vi "test Import Same Module Different Configuration.vi"(8 "error in (no error)":errorcluster, 11 "TestCase in":refnum<class "SLSC Switch Import Unit Tests.lvclass">) -> (0 "error out":errorcluster, 3 "TestCase out":refnum<class "SLSC Switch Import Unit Tests.lvclass">)   [LabVIEW 2017, in "SLSC Switch Import Unit Tests.lvclass"]
uses:
  SLSC Switch Import Unit Tests.lvclass
  Shared/Endpoint Configuration Cluster.ctl
  Shared/Endpoint Configuration Enum.ctl
  Scripting/Properties/SLSC Switch All Properties.ctl
  <vilib>/addons/_JKI Toolkits/VI Tester/TestCase.llb/TestCase.lvclass
  Shared/SLSC Switch Shared.lvlib
  Scripting/SLSC Switch Scripting.lvlib
  C:/Program Files (x86)/National Instruments/LabVIEW 2017/vi.lib/addons/_JKI Toolkits/VI Tester/TestCase.llb/TestCase.lvclass
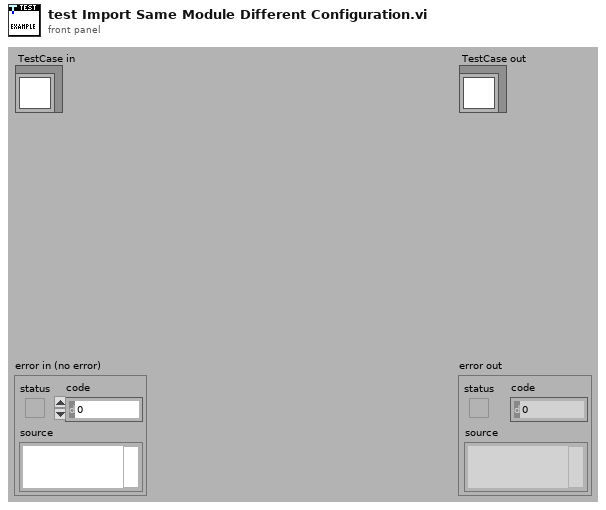
[diagram p1: front panel]
types:
  T1 = typedef "SLSC Switch Scripting.lvlib/SLSC Switch All Properties.ctl" = cluster{"Product Name":string, "Topology":string, "Switches JSON":string, "Description":string}
  T2 = typedef "SLSC Switch Shared.lvlib/Endpoint Configuration Cluster.ctl" = cluster{"Endpoint":string, "Configuration":T3}
  T3 = typedef "SLSC Switch Shared.lvlib/Endpoint Configuration Enum.ctl" = enum16{"Load", "Source", "Configuration"}
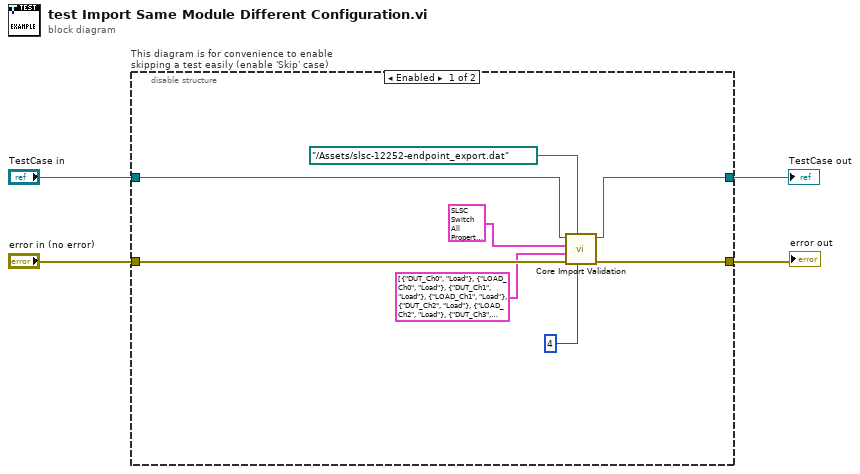
[diagram p0: block diagram]
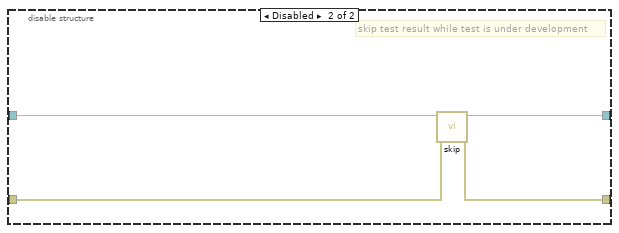
[diagram p2: hidden frame]
diagram:
  n1 = disable-structure "This diagram is for convenience to enable skipping a test easily (enable 'Skip' case)" shown="Enabled" {
    disable-tunnel: "TestCase in" -> [w8 w16]
    disable-tunnel: [w7 w14] -> w1
    disable-tunnel: [w6 w15] -> w3
    disable-tunnel: "error in (no error)" -> [w12 w13]
    frame Enabled {
      n2 = call "Core Import Validation.vi"("Slot Number"=u32 4 ("slot number"), "File to Import"=path "../Assets/slsc-12252-endpoint_export.dat" ("Path"), "error in (no error)"=w12, "Endpoint Configurations"=T2[] [{"Endpoint"="DUT_Ch0", "Configuration"=enum."Load"}, {"Endpoint"="LOAD_Ch0", "Configuration"=enum."Load"}, {"Endpoint"="DUT_Ch1", "Configuration"=enum."Load"}, {"Endpoint"="LOAD_Ch1", "Configuration"=enum."Load"}, {"Endpoint"="DUT_Ch2", "Configuration"=enum."Load"}, {"Endpoint"="LOAD_Ch2", "Configuration"=enum."Load"}, {"Endpoint"="DUT_Ch3", "Configuration"=enum."Load"}, {"Endpoint"="LOAD_Ch3", "Configuration"=enum."Load"}, {"Endpoint"="DUT_Ch4", "Configuration"=enum."Load"}, {"Endpoint"="LOAD_Ch4", "Configuration"=enum."Load"}, {"Endpoint"="DUT_Ch5", "Configuration"=enum."Load"}, {"Endpoint"="LOAD_Ch5", "Configuration"=enum."Load"}, {"Endpoint"="DUT_Ch6", "Configuration"=enum."Load"}, {"Endpoint"="LOAD_Ch6", "Configuration"=enum."Load"}, {"Endpoint"="DUT_Ch7", "Configuration"=enum."Load"}, {"Endpoint"="LOAD_Ch7", "Configuration"=enum."Load"}, {"Endpoint"="BusA", "Configuration"=enum."Source"}, {"Endpoint"="BusB", "Configuration"=enum."Configuration"}] ("All Endpoint Configurations"), "Switch Properties"=T1 {"Product Name"="SLSC-12252", "Topology"="NI12252_topology", "Switches JSON"="{\"switchesSpecVersion\":1,\"switchesSpecOldestCompatibleVersion\":1,\"relays\":[{\"name\":\"Ch0\",\"actions\":[{\"type\":\"property\",\"resource\":\"Channel_0\",\"value\":\"NI.FIU.Preset.Load\"},{\"type\":\"command\",\"resource\":\"\",\"value\":\"NI.FIU.Update\"}]},{\"name\":\"Ch1\",\"actions\":[{\"type\":\"property\",\"resource\":\"Channel_1\",\"value\":\"NI.FIU.Preset.Load\"},{\"type\":\"command\",\"resource\":\"\",\"value\":\"NI.FIU.Update\"}]},{\"name\":\"Ch2\",\"actions\":[{\"type\":\"property\",\"resource\":\"Channel_2\",\"value\":\"NI.FIU.Preset.Load\"},{\"type\":\"command\",\"resource\":\"\",\"value\":\"NI.FIU.Update\"}]},{\"name\":\"Ch3\",\"actions\":[{\"type\":\"property\",\"resource\":\"Channel_3\",\"value\":\"NI.FIU.Preset.Load\"},{\"type\":\"command\",\"resource\":\"\",\"value\":\"NI.FIU.Update\"}]},{\"name\":\"Ch4\",\"actions\":[{\"type\":\"property\",\"resource\":\"Channel_4\",\"value\":\"NI.FIU.Preset.Load\"},{\"type\":\"command\",\"resource\":\"\",\"value\":\"NI.FIU.Update\"}]},{\"name\":\"Ch5\",\"actions\":[{\"type\":\"property\",\"resource\":\"Channel_5\",\"value\":\"NI.FIU.Preset.Load\"},{\"type\":\"command\",\"resource\":\"\",\"value\":\"NI.FIU.Update\"}]},{\"name\":\"Ch6\",\"actions\":[{\"type\":\"property\",\"resource\":\"Channel_6\",\"value\":\"NI.FIU.Preset.Load\"},{\"type\":\"command\",\"resource\":\"\",\"value\":\"NI.FIU.Update\"}]},{\"name\":\"Ch7\",\"actions\":[{\"type\":\"property\",\"resource\":\"Channel_7\",\"value\":\"NI.FIU.Preset.Load\"},{\"type\":\"command\",\"resource\":\"\",\"value\":\"NI.FIU.Update\"}]},{\"name\":\"Ch0_Ch1\",\"actions\":[{\"type\":\"property\",\"resource\":\"ChannelPair_0\",\"value\":\"NI.FIU.Preset.InterChannel\"},{\"type\":\"command\",\"resource\":\"\",\"value\":\"NI.FIU.Update\"}]},{\"name\":\"Ch2_Ch3\",\"actions\":[{\"type\":\"property\",\"resource\":\"ChannelPair_1\",\"value\":\"NI.FIU.Preset.InterChannel\"},{\"type\":\"command\",\"resource\":\"\",\"value\":\"NI.FIU.Update\"}]},{\"name\":\"Ch4_Ch5\",\"actions\":[{\"type\":\"property\",\"resource\":\"ChannelPair_2\",\"value\":\"NI.FIU.Preset.InterChannel\"},{\"type\":\"command\",\"resource\":\"\",\"value\":\"NI.FIU.Update\"}]},{\"name\":\"Ch6_Ch7\",\"actions\":[{\"type\":\"property\",\"resource\":\"ChannelPair_3\",\"value\":\"NI.FIU.Preset.InterChannel\"},{\"type\":\"command\",\"resource\":\"\",\"value\":\"NI.FIU.Update\"}]}],\"multiStateRelays\":[{\"name\":\"Ch0_Bus\",\"relays\":[{\"name\":\"Ch0_BusA\",\"actions\":[{\"type\":\"property\",\"resource\":\"Channel_0\",\"value\":\"NI.FIU.Preset.BusSource\",\"close\":1},{\"type\":\"command\",\"resource\":\"\",\"value\":\"NI.FIU.Update\"}]},{\"name\":\"Ch0_BusB\",\"actions\":[{\"type\":\"property\",\"resource\":\"Channel_0\",\"value\":\"NI.FIU.Preset.BusSource\",\"close\":2},{\"type\":\"command\",\"resource\":\"\",\"value\":\"NI.FIU.Update\"}]}]},{\"name\":\"Ch1_Bus\",\"relays\":[{\"name\":\"Ch1_BusA\",\"actions\":[{\"type\":\"property\",\"resource\":\"Channel_1\",\"value\":\"NI.FIU.Preset.BusSource\",\"close\":1},{\"type\":\"command\",\"resource\":\"\",\"value\":\"NI.FIU.Update\"}]},{\"name\":\"Ch1_BusB\",\"actions\":[{\"type\":\"property\",\"resource\":\"Channel_1\",\"value\":\"NI.FIU.Preset.BusSource\",\"close\":2},{\"type\":\"command\",\"resource\":\"\",\"value\":\"NI.FIU.Update\"}]}]},{\"name\":\"Ch2_Bus\",\"relays\":[{\"name\":\"Ch2_BusA\",\"actions\":[{\"type\":\"property\",\"resource\":\"Channel_2\",\"value\":\"NI.FIU.Preset.BusSource\",\"close\":1},{\"type\":\"command\",\"resource\":\"\",\"value\":\"NI.FIU.Update\"}]},{\"name\":\"Ch2_BusB\",\"actions\":[{\"type\":\"property\",\"resource\":\"Channel_2\",\"value\":\"NI.FIU.Preset.BusSource\",\"close\":2},{\"type\":\"command\",\"resource\":\"\",\"value\":\"NI.FIU.Update\"}]}]},{\"name\":\"Ch3_Bus\",\"relays\":[{\"name\":\"Ch3_BusA\",\"actions\":[{\"type\":\"property\",\"resource\":\"Channel_3\",\"value\":\"NI.FIU.Preset.BusSource\",\"close\":1},{\"type\":\"command\",\"resource\":\"\",\"value\":\"NI.FIU.Update\"}]},{\"name\":\"Ch3_BusB\",\"actions\":[{\"type\":\"property\",\"resource\":\"Channel_3\",\"value\":\"NI.FIU.Preset.BusSource\",\"close\":2},{\"type\":\"command\",\"resource\":\"\",\"value\":\"NI.FIU.Update\"}]}]},{\"name\":\"Ch4_Bus\",\"relays\":[{\"name\":\"Ch4_BusA\",\"actions\":[{\"type\":\"property\",\"resource\":\"Channel_4\",\"value\":\"NI.FIU.Preset.BusSource\",\"close\":1},{\"type\":\"command\",\"resource\":\"\",\"value\":\"NI.FIU.Update\"}]},{\"name\":\"Ch4_BusB\",\"actions\":[{\"type\":\"property\",\"resource\":\"Channel_4\",\"value\":\"NI.FIU.Preset.BusSource\",\"close\":2},{\"type\":\"command\",\"resource\":\"\",\"value\":\"NI.FIU.Update\"}]}]},{\"name\":\"Ch5_Bus\",\"relays\":[{\"name\":\"Ch5_BusA\",\"actions\":[{\"type\":\"property\",\"resource\":\"Channel_5\",\"value\":\"NI.FIU.Preset.BusSource\",\"close\":1},{\"type\":\"command\",\"resource\":\"\",\"value\":\"NI.FIU.Update\"}]},{\"name\":\"Ch5_BusB\",\"actions\":[{\"type\":\"property\",\"resource\":\"Channel_5\",\"value\":\"NI.FIU.Preset.BusSource\",\"close\":2},{\"type\":\"command\",\"resource\":\"\",\"value\":\"NI.FIU.Update\"}]}]},{\"name\":\"Ch6_Bus\",\"relays\":[{\"name\":\"Ch6_BusA\",\"actions\":[{\"type\":\"property\",\"resource\":\"Channel_6\",\"value\":\"NI.FIU.Preset.BusSource\",\"close\":1},{\"type\":\"command\",\"resource\":\"\",\"value\":\"NI.FIU.Update\"}]},{\"name\":\"Ch6_BusB\",\"actions\":[{\"type\":\"property\",\"resource\":\"Channel_6\",\"value\":\"NI.FIU.Preset.BusSource\",\"close\":2},{\"type\":\"command\",\"resource\":\"\",\"value\":\"NI.FIU.Update\"}]}]},{\"name\":\"Ch7_Bus\",\"relays\":[{\"name\":\"Ch7_BusA\",\"actions\":[{\"type\":\"property\",\"resource\":\"Channel_7\",\"value\":\"NI.FIU.Preset.BusSource\",\"close\":1},{\"type\":\"command\",\"resource\":\"\",\"value\":\"NI.FIU.Update\"}]},{\"name\":\"Ch7_BusB\",\"actions\":[{\"type\":\"property\",\"resource\":\"Channel_7\",\"value\":\"NI.FIU.Preset.BusSource\",\"close\":2},{\"type\":\"command\",\"resource\":\"\",\"value\":\"NI.FIU.Update\"}]}]}],\"topologies\":[{\"name\":\"NI12252_topology\",\"initialState\":{\"open\":[\"Ch0\",\"Ch0_BusA\",\"Ch0_BusB\",\"Ch1\",\"Ch1_BusA\",\"Ch1_BusB\",\"Ch2\",\"Ch2_BusA\",\"Ch2_BusB\",\"Ch3\",\"Ch3_BusA\",\"Ch3_BusB\",\"Ch4\",\"Ch4_BusA\",\"Ch4_BusB\",\"Ch5\",\"Ch5_BusA\",\"Ch5_BusB\",\"Ch6\",\"Ch6_BusA\",\"Ch6_BusB\",\"Ch7\",\"Ch7_BusA\",\"Ch7_BusB\",\"Ch0_Ch1\",\"Ch2_Ch3\",\"Ch4_Ch5\",\"Ch6_Ch7\"],\"close\":[]},\"channelList\":{\"names\":[\"DUT_Ch0\",\"LOAD_Ch0\",\"DUT_Ch1\",\"LOAD_Ch1\",\"DUT_Ch2\",\"LOAD_Ch2\",\"DUT_Ch3\",\"LOAD_Ch3\",\"DUT_Ch4\",\"LOAD_Ch4\",\"DUT_Ch5\",\"LOAD_Ch5\",\"DUT_Ch6\",\"LOAD_Ch6\",\"DUT_Ch7\",\"LOAD_Ch7\",\"BusA\",\"BusB\"]},\"connectionList\":[{\"src\":\"DUT_Ch0\",\"dest\":\"LOAD_Ch0\",\"relays\":[\"Ch0\"]},{\"src\":\"DUT_Ch0\",\"dest\":\"BusA\",\"relays\":[\"Ch0_BusA\"]},{\"src\":\"DUT_Ch0\",\"dest\":\"BusB\",\"relays\":[\"Ch0_BusB\"]},{\"src\":\"DUT_Ch1\",\"dest\":\"LOAD_Ch1\",\"relays\":[\"Ch1\"]},{\"src\":\"DUT_Ch1\",\"dest\":\"BusA\",\"relays\":[\"Ch1_BusA\"]},{\"src\":\"DUT_Ch1\",\"dest\":\"BusB\",\"relays\":[\"Ch1_BusB\"]},{\"src\":\"DUT_Ch2\",\"dest\":\"LOAD_Ch2\",\"relays\":[\"Ch2\"]},{\"src\":\"DUT_Ch2\",\"dest\":\"BusA\",\"relays\":[\"Ch2_BusA\"]},{\"src\":\"DUT_Ch2\",\"dest\":\"BusB\",\"relays\":[\"Ch2_BusB\"]},{\"src\":\"DUT_Ch3\",\"dest\":\"LOAD_Ch3\",\"relays\":[\"Ch3\"]},{\"src\":\"DUT_Ch3\",\"dest\":\"BusA\",\"relays\":[\"Ch3_BusA\"]},{\"src\":\"DUT_Ch3\",\"dest\":\"BusB\",\"relays\":[\"Ch3_BusB\"]},{\"src\":\"DUT_Ch4\",\"dest\":\"LOAD_Ch4\",\"relays\":[\"Ch4\"]},{\"src\":\"DUT_Ch4\",\"dest\":\"BusA\",\"relays\":[\"Ch4_BusA\"]},{\"src\":\"DUT_Ch4\",\"dest\":\"BusB\",\"relays\":[\"Ch4_BusB\"]},{\"src\":\"DUT_Ch5\",\"dest\":\"LOAD_Ch5\",\"relays\":[\"Ch5\"]},{\"src\":\"DUT_Ch5\",\"dest\":\"BusA\",\"relays\":[\"Ch5_BusA\"]},{\"src\":\"DUT_Ch5\",\"dest\":\"BusB\",\"relays\":[\"Ch5_BusB\"]},{\"src\":\"DUT_Ch6\",\"dest\":\"LOAD_Ch6\",\"relays\":[\"Ch6\"]},{\"src\":\"DUT_Ch6\",\"dest\":\"BusA\",\"relays\":[\"Ch6_BusA\"]},{\"src\":\"DUT_Ch6\",\"dest\":\"BusB\",\"relays\":[\"Ch6_BusB\"]},{\"src\":\"DUT_Ch7\",\"dest\":\"LOAD_Ch7\",\"relays\":[\"Ch7\"]},{\"src\":\"DUT_Ch7\",\"dest\":\"BusA\",\"relays\":[\"Ch7_BusA\"]},{\"src\":\"DUT_Ch7\",\"dest\":\"BusB\",\"relays\":[\"Ch7_BusB\"]},{\"src\":\"DUT_Ch0\",\"dest\":\"DUT_Ch1\",\"relays\":[\"Ch0_Ch1\"]},{\"src\":\"DUT_Ch2\",\"dest\":\"DUT_Ch3\",\"relays\":[\"Ch2_Ch3\"]},{\"src\":\"DUT_Ch4\",\"dest\":\"DUT_Ch5\",\"relays\":[\"Ch4_Ch5\"]},{\"src\":\"DUT_Ch6\",\"dest\":\"DUT_Ch7\",\"relays\":[\"Ch6_Ch7\"]}],\"muxList\":[{\"src\":\"DUT_Ch0\",\"dest\":[\"BusA\",\"BusB\"]},{\"src\":\"DUT_Ch1\",\"dest\":[\"BusA\",\"BusB\"]},{\"src\":\"DUT_Ch2\",\"dest\":[\"BusA\",\"BusB\"]},{\"src\":\"DUT_Ch3\",\"dest\":[\"BusA\",\"BusB\"]},{\"src\":\"DUT_Ch4\",\"dest\":[\"BusA\",\"BusB\"]},{\"src\":\"DUT_Ch5\",\"dest\":[\"BusA\",\"BusB\"]},{\"src\":\"DUT_Ch6\",\"dest\":[\"BusA\",\"BusB\"]},{\"src\":\"DUT_Ch7\",\"dest\":[\"BusA\",\"BusB\"]}]}]}", "Description"=""} ("SLSC Switch All Properties"), "SLSC Switch Import Unit Tests in"=w8) -> ("error out"=w6:errorcluster, "SLSC Switch Import Unit Tests out"=w7:refnum<class "SLSC Switch Import Unit Tests.lvclass">)  [unwired: 4 in]
    }
    frame Disabled {
      # "skip test result while test is under development"
      n3 = call <vilib>:"skip.vi"("error in (no error)"=w13, "TestCase in"=w16) -> ("error out"=w15:errorcluster, "TestCase out"=w14:refnum<class "SLSC Switch Import Unit Tests.lvclass">)  [unwired: 8 in]
    }
  }
  "error out" <- w3
  "TestCase out" <- w1
